vi "final_UI.vi"() -> ()   [LabVIEW 2020]
panel:
  in  "VISA resource name":refnum<visa-resource-name>
  in  "Table Control":string[][](table)
  out "humidity":dbl(graph)
  out "Temp":dbl(graph)
  out "humidity":dbl(knob) scale=0.0..100.0
  out "Temp":dbl(slide) scale=0.0..50.0
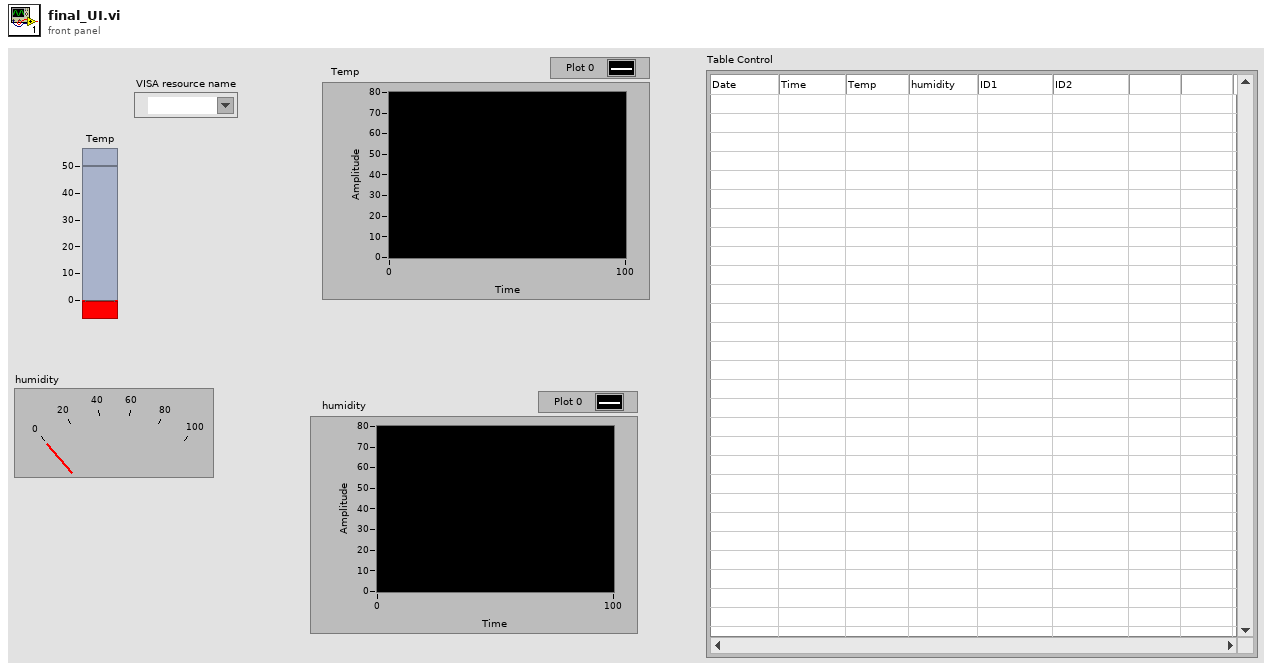
[diagram p1: front panel]
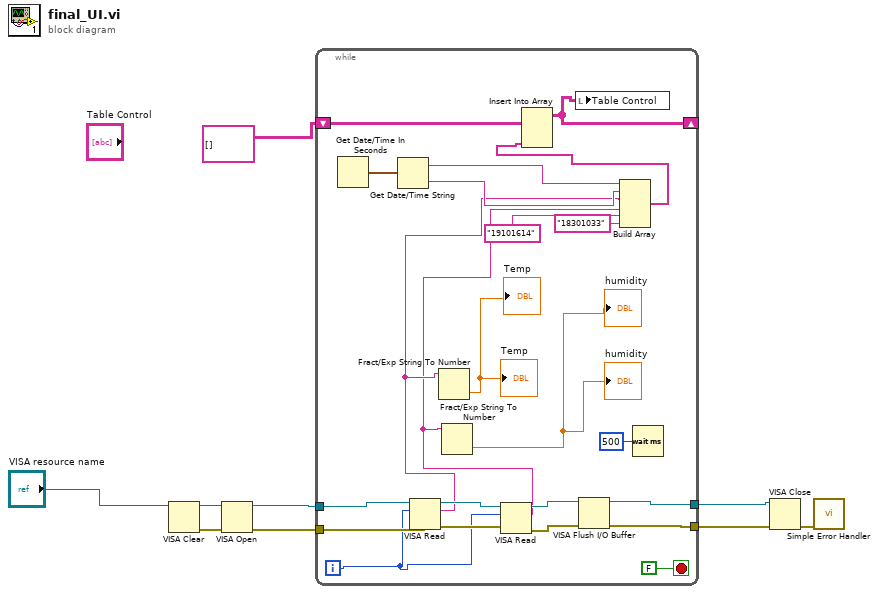
[diagram p0: block diagram]
diagram:
  n1 = VISA Clear(VISA resource name="VISA resource name") -> (VISA resource name out=w8:refnum<visa-resource-name>, error out=w9:errorcluster)  [unwired: 1 in]
  n2 = VISA Open(error in (no error)=w9, VISA resource name=w8) -> (VISA resource name=w6:refnum<visa-resource-name>, error out=w5:errorcluster)  [unwired: 3 in]
  n3 = while {
    tunnel: w6 -> [w32]
    tunnel: w5 -> [w29]
    tunnel: [w26] -> w4
    tunnel: [w25] -> w3
    shift-right: [w21] -> _
    shift-left: string[][] [] -> [w22]
    i -> [w24]
    stop <- FALSE stop-if-true
    n4 = Get Date/Time In Seconds() -> (seconds since 1Jan1904=w18:timestamp)
    n5 = Get Date/Time String(seconds (now)=w18) -> (date string=w17:string, time string=w16:string)  [unwired: 2 in]
    n6 = VISA Read(VISA resource name=w32, byte count=w24, error in (no error)=w29) -> (VISA resource name out=w31:refnum<visa-resource-name>, read buffer=w15:string, error out=w28:errorcluster)  [unwired: 1 out]
    n7 = Fract/Exp String To Number(string=w15) -> (number=→"Temp" →"Temp":dbl)  [unwired: 3 in, 1 out]
    n8 = VISA Read(VISA resource name=w31, byte count=w24, error in (no error)=w28) -> (VISA resource name out=w30:refnum<visa-resource-name>, read buffer=w14:string, error out=w27:errorcluster)  [unwired: 1 out]
    n9 = Fract/Exp String To Number(string=w14) -> (number=→"humidity" →"humidity":dbl)  [unwired: 3 in, 1 out]
    n10 = VISA Flush I/O Buffer(VISA resource name=w30, error in (no error)=w27) -> (VISA resource name out=w26:refnum<visa-resource-name>, error out=w25:errorcluster)  [unwired: 1 in]
    n11 = Build Array(w17, w16, w15, w14, "19101614" ("element"), "18301033" ("element")) -> (w11:string[])
    n12 = Insert Into Array(array=w22, new element=w11) -> (w21:string[][])  [unwired: 2 in]
    n13 = local write "Table Control"(w21) -> ()
    n14 = Wait (ms)(milliseconds to wait=u32 500) -> ()  [unwired: 1 out]
  }
  n15 = VISA Close(VISA resource name=w4, error in (no error)=w3) -> (error out=w7:errorcluster)
  n16 = call <vilib>:"Simple Error Handler.vi"("error in (no error)"=w7) -> ()  [unwired: 4 in, 5 out]
